vi "CreateWaveData.vi"(8 "error in (no error)":errorcluster, 11 "Sine in":refnum<class "Sine.lvclass">) -> (0 "error out":errorcluster, 2 "signal out":waveform(dbl), 3 "Sine out":refnum<class "Sine.lvclass">)   [LabVIEW 2021, in "Sine.lvclass"]
uses:
  Sine.lvclass
  <vilib>/measure/NI_MABase.lvlib
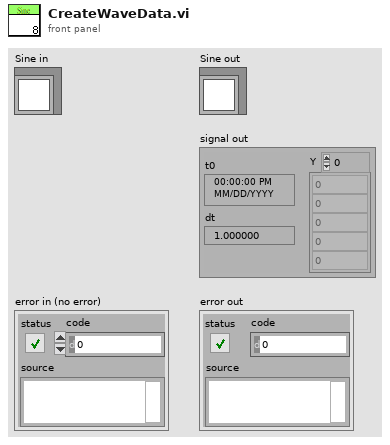
[diagram p1: front panel]
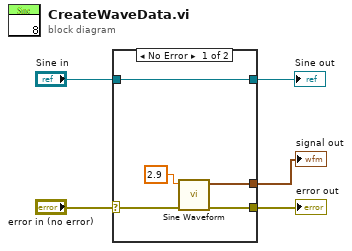
[diagram p0: block diagram]
diagram:
  n1 = case shown="No Error" "error in (no error)" {
    selector: "error in (no error)" -> [w8 w11]
    tunnel: [w10 w11] -> w5
    tunnel: [w9 _] -> w4
    tunnel: [w7 w12] -> w3
    tunnel: "Sine in" -> [w7 w12]
    frame No Error {
      n2 = call <vilib>:"Sine Waveform.vi"("error in (no error)"=w8, "frequency"=2.9) -> ("error out"=w10:errorcluster, "signal out"=w9:waveform(dbl))  [unwired: 8 in]
    }
    frame Error {
    }
  }
  "Sine out" <- w3
  "signal out" <- w4
  "error out" <- w5
